vi "ScalarVariantToData.vi"(8 "error in (no error)":errorcluster, 10 "type":T1, 11 "Variant":variant) -> (0 "error out":errorcluster, 2 "Type":string, 3 "Value":string)   [LabVIEW 2019, in "BlueVariantView.lvlib"]
uses:
  BlueVariantView.lvlib
  <vilib>/Utility/Data Type/Type Definitions/Data Type.ctl
  <vilib>/Utility/error.llb/Error Cluster From Error Code.vi
  <vilib>/ErrorRing/Error Ring.xnode
  <vilib>/Utility/Data Type/NI_Data Type.lvlib
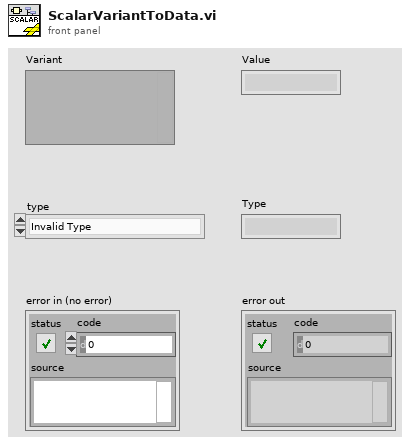
[diagram p1: front panel]
types:
  T1 = typedef "NI_Data Type.lvlib/Data Type.ctl" = enum8{"Invalid Type", "Void", "I8", "I16", "I32", "I64", "U8", "U16", "U32", "U64", "Single Float", "Double Float", "Extended Float", "Single Complex", "Double Complex", "Extended Complex", "Enum U8", "Enum U16", "Enum U32", "Enum U64", "Single Float With Unit", "Double Float With Unit", "Extended Float With Unit", "Single Complex with Unit", "Double Complex with Unit", "Extended Complex with Unit", "Boolean", "String", "Path", "Picture", "Tag", "Array", "Cluster", "Variant", "LV Variant", "Waveform", "Timestamp", "Digital Waveform", "Digital Data", "ExpressData", "Refnum", "External Data", "VI", "Poly VI", "LabVIEW Class Instance", "Fixed Point", "Set Collection", "Map Collection"}
  T2 = typedef "Physical Units__ogtk.ctl" = cluster{"Base Units":enum16{"radian", "steradian", "second", "meter", "kilogram", "ampere", "kelvin", "mole", "candela"}, "Exponent":i16}
  T3 = enum16{"radian", "steradian", "second", "meter", "kilogram", "ampere", "kelvin", "mole", "candela"}
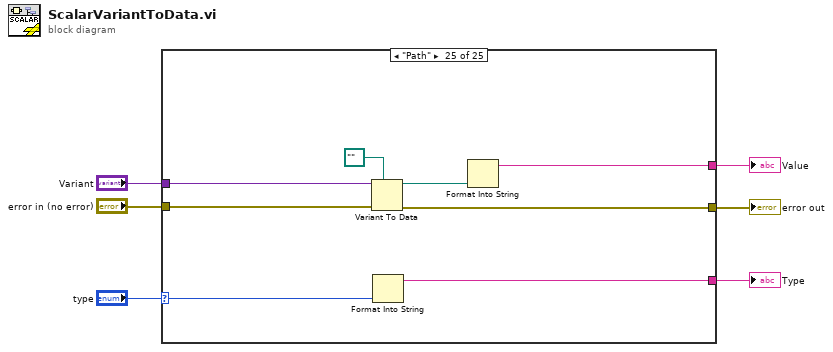
[diagram p0: block diagram]
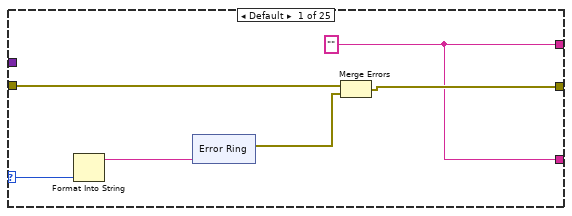
[diagram p2: hidden frame]
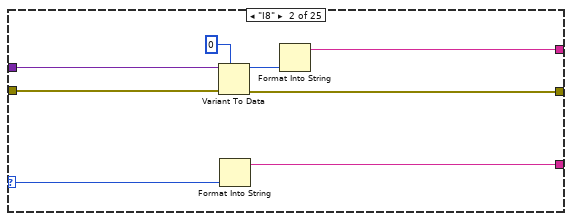
[diagram p3: hidden frame]
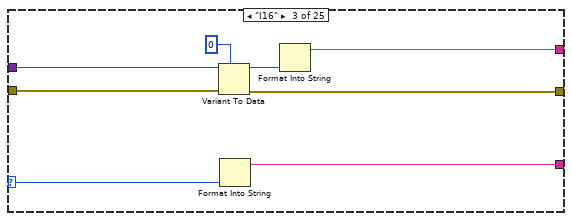
[diagram p4: hidden frame]
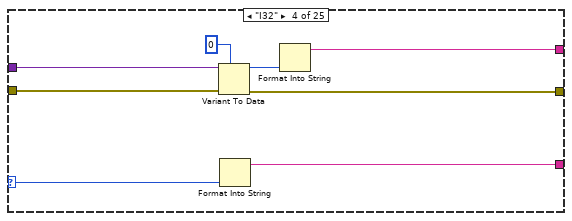
[diagram p5: hidden frame]
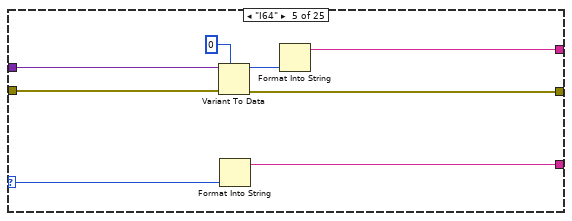
[diagram p6: hidden frame]
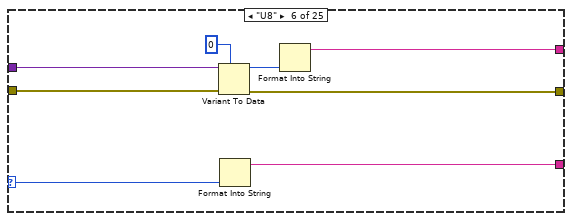
[diagram p7: hidden frame]
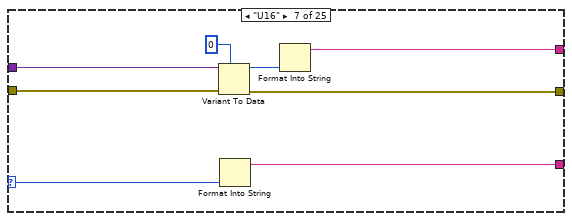
[diagram p8: hidden frame]
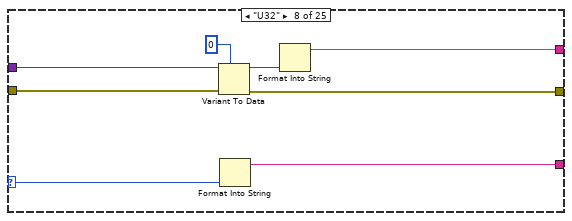
[diagram p9: hidden frame]
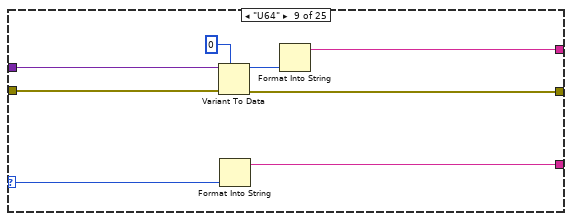
[diagram p10: hidden frame]
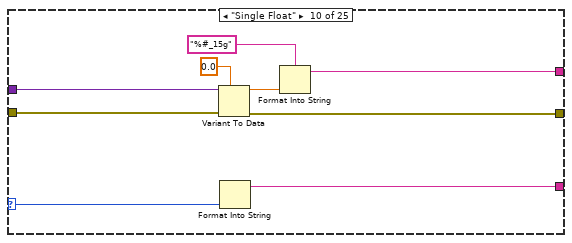
[diagram p11: hidden frame]
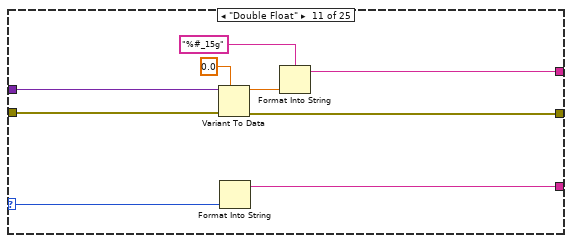
[diagram p12: hidden frame]
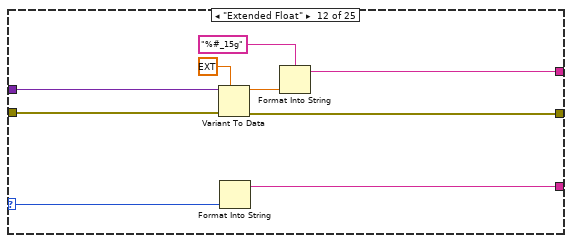
[diagram p13: hidden frame]
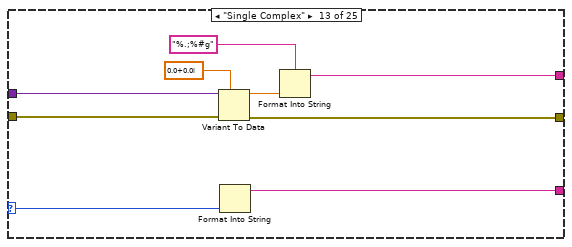
[diagram p14: hidden frame]
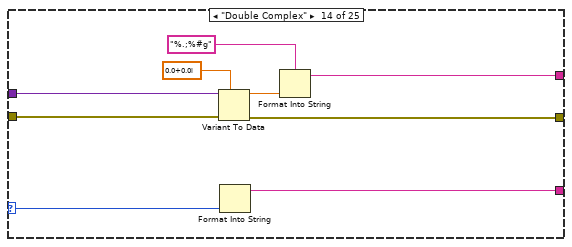
[diagram p15: hidden frame]
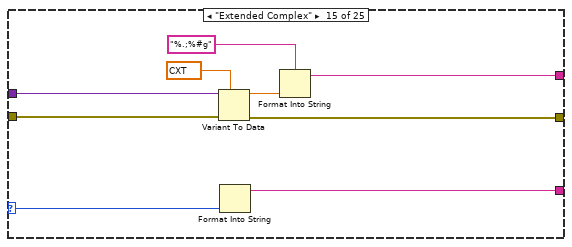
[diagram p16: hidden frame]
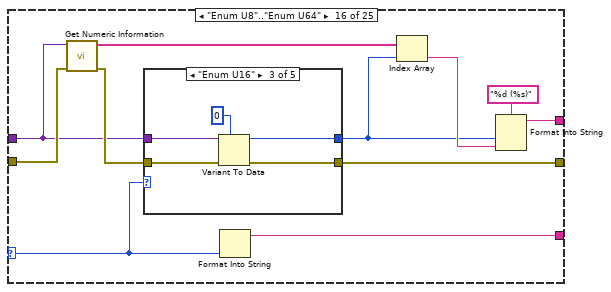
[diagram p17: hidden frame]
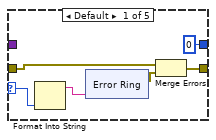
[diagram p18: hidden frame]
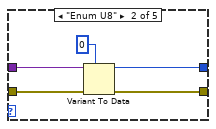
[diagram p19: hidden frame]
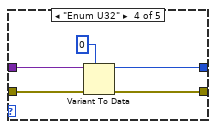
[diagram p20: hidden frame]
diagram:
  n1 = case shown="\"Path\"" "type" {
    selector: "type" -> [w12 w23 w31 w39 w47 w55 w63 w71 w79 w88 w97 w106 w115 w124 w133 w142 w192 w205 w218 w231 w244 w257 w264 w271 w279]
    tunnel: "Variant" -> [_ w27 w35 w43 w51 w59 w67 w75 w83 w92 w101 w110 w119 w128 w137 w143 w185 w198 w211 w224 w237 w250 w267 w274 w282]
    tunnel: "error in (no error)" -> [w10 w26 w34 w42 w50 w58 w66 w74 w82 w91 w100 w109 w118 w127 w136 w145 w187 w200 w213 w226 w239 w252 w266 w273 w281]
    tunnel: [w8 w24 w32 w40 w48 w56 w64 w72 w80 w89 w98 w107 w116 w125 w134 w148 w193 w206 w219 w232 w245 w258 w265 w272 w280] -> w4
    tunnel: [w7 w22 w30 w38 w46 w54 w62 w70 w78 w87 w96 w105 w114 w123 w132 w147 w191 w204 w217 w230 w243 w256 w263 w270 w278] -> w2
    tunnel: [w7 w20 w28 w36 w44 w52 w60 w68 w76 w85 w94 w103 w112 w121 w130 w146 w189 w202 w215 w228 w241 w254 w261 w268 w275] -> w1
    frame Default {
      w7 = ""
      n2 = Format Into String(w12) -> (resulting string=w11:string)  [unwired: 3 in, 1 out]
      n3 = xnode "Error Ring"("parameter 0"=w11) -> ("error out"=w9:errorcluster)
      n4 = Merge Errors(w10, w9) -> (w8:errorcluster)
    }
    frame "I8" {
      n5 = Variant To Data(error in=w26, type=i8 0, Variant=w27) -> (data=w21:i8, error out=w24:errorcluster)
      n6 = Format Into String(w23) -> (resulting string=w22:string)  [unwired: 3 in, 1 out]
      n7 = Format Into String(w21) -> (resulting string=w20:string)  [unwired: 3 in, 1 out]
    }
    frame "I16" {
      n8 = Variant To Data(error in=w34, type=i16 0, Variant=w35) -> (data=w29:i16, error out=w32:errorcluster)
      n9 = Format Into String(w31) -> (resulting string=w30:string)  [unwired: 3 in, 1 out]
      n10 = Format Into String(w29) -> (resulting string=w28:string)  [unwired: 3 in, 1 out]
    }
    frame "I32" {
      n11 = Variant To Data(error in=w42, type=0, Variant=w43) -> (data=w37:i32, error out=w40:errorcluster)
      n12 = Format Into String(w39) -> (resulting string=w38:string)  [unwired: 3 in, 1 out]
      n13 = Format Into String(w37) -> (resulting string=w36:string)  [unwired: 3 in, 1 out]
    }
    frame "I64" {
      n14 = Variant To Data(error in=w50, type=i64 0, Variant=w51) -> (data=w45:i64, error out=w48:errorcluster)
      n15 = Format Into String(w47) -> (resulting string=w46:string)  [unwired: 3 in, 1 out]
      n16 = Format Into String(w45) -> (resulting string=w44:string)  [unwired: 3 in, 1 out]
    }
    frame "U8" {
      n17 = Variant To Data(error in=w58, type=u8 0, Variant=w59) -> (data=w53:u8, error out=w56:errorcluster)
      n18 = Format Into String(w55) -> (resulting string=w54:string)  [unwired: 3 in, 1 out]
      n19 = Format Into String(w53) -> (resulting string=w52:string)  [unwired: 3 in, 1 out]
    }
    frame "U16" {
      n20 = Variant To Data(error in=w66, type=u16 0, Variant=w67) -> (data=w61:u16, error out=w64:errorcluster)
      n21 = Format Into String(w63) -> (resulting string=w62:string)  [unwired: 3 in, 1 out]
      n22 = Format Into String(w61) -> (resulting string=w60:string)  [unwired: 3 in, 1 out]
    }
    frame "U32" {
      n23 = Variant To Data(error in=w74, type=u32 0, Variant=w75) -> (data=w69:u32, error out=w72:errorcluster)
      n24 = Format Into String(w71) -> (resulting string=w70:string)  [unwired: 3 in, 1 out]
      n25 = Format Into String(w69) -> (resulting string=w68:string)  [unwired: 3 in, 1 out]
    }
    frame "U64" {
      n26 = Variant To Data(error in=w82, type=u64 0, Variant=w83) -> (data=w77:u64, error out=w80:errorcluster)
      n27 = Format Into String(w79) -> (resulting string=w78:string)  [unwired: 3 in, 1 out]
      n28 = Format Into String(w77) -> (resulting string=w76:string)  [unwired: 3 in, 1 out]
    }
    frame "Single Float" {
      n29 = Variant To Data(error in=w91, type=sgl 0.0, Variant=w92) -> (data=w86:sgl, error out=w89:errorcluster)
      n30 = Format Into String(w88) -> (resulting string=w87:string)  [unwired: 3 in, 1 out]
      n31 = Format Into String(format string="%#_15g", w86) -> (resulting string=w85:string)  [unwired: 2 in, 1 out]
    }
    frame "Double Float" {
      n32 = Variant To Data(error in=w100, type=0.0, Variant=w101) -> (data=w95:dbl, error out=w98:errorcluster)
      n33 = Format Into String(w97) -> (resulting string=w96:string)  [unwired: 3 in, 1 out]
      n34 = Format Into String(format string="%#_15g", w95) -> (resulting string=w94:string)  [unwired: 2 in, 1 out]
    }
    frame "Extended Float" {
      n35 = Variant To Data(error in=w109, type=ext 0.0, Variant=w110) -> (data=w104:ext, error out=w107:errorcluster)
      n36 = Format Into String(w106) -> (resulting string=w105:string)  [unwired: 3 in, 1 out]
      n37 = Format Into String(format string="%#_15g", w104) -> (resulting string=w103:string)  [unwired: 2 in, 1 out]
    }
    frame "Single Complex" {
      n38 = Variant To Data(error in=w118, type=csg 0.0+0.0i, Variant=w119) -> (data=w113:csg, error out=w116:errorcluster)
      n39 = Format Into String(w115) -> (resulting string=w114:string)  [unwired: 3 in, 1 out]
      n40 = Format Into String(format string="%.;%#g", w113) -> (resulting string=w112:string)  [unwired: 2 in, 1 out]
    }
    frame "Double Complex" {
      n41 = Variant To Data(error in=w127, type=cdb 0.0+0.0i, Variant=w128) -> (data=w122:cdb, error out=w125:errorcluster)
      n42 = Format Into String(w124) -> (resulting string=w123:string)  [unwired: 3 in, 1 out]
      n43 = Format Into String(format string="%.;%#g", w122) -> (resulting string=w121:string)  [unwired: 2 in, 1 out]
    }
    frame "Extended Complex" {
      n44 = Variant To Data(error in=w136, type=cxt 0.0+0.0i, Variant=w137) -> (data=w131:cxt, error out=w134:errorcluster)
      n45 = Format Into String(w133) -> (resulting string=w132:string)  [unwired: 3 in, 1 out]
      n46 = Format Into String(format string="%.;%#g", w131) -> (resulting string=w130:string)  [unwired: 2 in, 1 out]
    }
    frame "Enum U8".."Enum U64" {
      n47 = call <vilib>:"Get Numeric Information.vi"("error in (no error)"=w145, "variant"=w143) -> ("error out"=w144:errorcluster, "enum names"=w141:string[])  [unwired: 6 in, 2 out]
      n48 = case shown="\"Enum U16\"" w142 {
        selector: w142 -> [w153 _ _ _ _]
        tunnel: [w150 w165 w170 w175 w180] -> w148
        tunnel: [u64 0 w164 w169 w174 w179] -> w138
        tunnel: w144 -> [w151 w163 w168 w173 w178]
        tunnel: w143 -> [_ w162 w167 w172 w177]
        frame Default {
          n49 = Format Into String(w153) -> (resulting string=w152:string)  [unwired: 3 in, 1 out]
          n50 = xnode "Error Ring"("parameter 0"=w152) -> ("error out"=w149:errorcluster)
          n51 = Merge Errors(w151, w149) -> (w150:errorcluster)
        }
        frame "Enum U8" {
          n52 = Variant To Data(error in=w163, type=u8 0, Variant=w162) -> (data=w164:u8, error out=w165:errorcluster)
        }
        frame "Enum U16" {
          n53 = Variant To Data(error in=w168, type=u16 0, Variant=w167) -> (data=w169:u16, error out=w170:errorcluster)
        }
        frame "Enum U32" {
          n54 = Variant To Data(error in=w173, type=u32 0, Variant=w172) -> (data=w174:u32, error out=w175:errorcluster)
        }
        frame "Enum U64" {
          n55 = Variant To Data(error in=w178, type=u64 0, Variant=w177) -> (data=w179:u64, error out=w180:errorcluster)
        }
      }
      n56 = Format Into String(w142) -> (resulting string=w147:string)  [unwired: 3 in, 1 out]
      n57 = Index Array(array=w141, index=w138) -> (element=w139:string)
      n58 = Format Into String(format string="%d (%s)", w138, w139) -> (resulting string=w146:string)  [unwired: 2 in, 1 out]
    }
    frame "Single Float With Unit" {
      n59 = call <userlib>:"Get Physical Units__ogtk.vi"("error in (no error)"=w187, "Float or Array of Floats"=w185) -> ("error out"=w186:errorcluster, "Physical Units"=w184:T2[])  [unwired: 8 in]
      n60 = Index Array(array=w184) -> (element=w183:T2)  [unwired: 1 in]
      n61 = Variant To Data(error in=w186, type=sgl 0.0, Variant=w185) -> (data=w190:sgl, error out=w193:errorcluster)
      n62 = Format Into String(w192) -> (resulting string=w191:string)  [unwired: 3 in, 1 out]
      n63 = Unbundle By Name(w183) -> ("Base Units"=w182:T3)
      n64 = Format Into String(format string="%#_15g (%s)", w190, w182) -> (resulting string=w189:string)  [unwired: 2 in, 1 out]
    }
    frame "Double Float With Unit" {
      n65 = call <userlib>:"Get Physical Units__ogtk.vi"("error in (no error)"=w200, "Float or Array of Floats"=w198) -> ("error out"=w199:errorcluster, "Physical Units"=w197:T2[])  [unwired: 8 in]
      n66 = Index Array(array=w197) -> (element=w196:T2)  [unwired: 1 in]
      n67 = Variant To Data(error in=w199, type=0.0, Variant=w198) -> (data=w203:dbl, error out=w206:errorcluster)
      n68 = Format Into String(w205) -> (resulting string=w204:string)  [unwired: 3 in, 1 out]
      n69 = Unbundle By Name(w196) -> ("Base Units"=w195:T3)
      n70 = Format Into String(format string="%#_15g (%s)", w203, w195) -> (resulting string=w202:string)  [unwired: 2 in, 1 out]
    }
    frame "Extended Float With Unit" {
      n71 = call <userlib>:"Get Physical Units__ogtk.vi"("error in (no error)"=w213, "Float or Array of Floats"=w211) -> ("error out"=w212:errorcluster, "Physical Units"=w210:T2[])  [unwired: 8 in]
      n72 = Index Array(array=w210) -> (element=w209:T2)  [unwired: 1 in]
      n73 = Variant To Data(error in=w212, type=ext 0.0, Variant=w211) -> (data=w216:ext, error out=w219:errorcluster)
      n74 = Format Into String(w218) -> (resulting string=w217:string)  [unwired: 3 in, 1 out]
      n75 = Unbundle By Name(w209) -> ("Base Units"=w208:T3)
      n76 = Format Into String(format string="%#_15g (%s)", w216, w208) -> (resulting string=w215:string)  [unwired: 2 in, 1 out]
    }
    frame "Single Complex with Unit" {
      n77 = call <userlib>:"Get Physical Units__ogtk.vi"("error in (no error)"=w226, "Float or Array of Floats"=w224) -> ("error out"=w225:errorcluster, "Physical Units"=w223:T2[])  [unwired: 8 in]
      n78 = Index Array(array=w223) -> (element=w222:T2)  [unwired: 1 in]
      n79 = Variant To Data(error in=w225, type=csg 0.0+0.0i, Variant=w224) -> (data=w229:csg, error out=w232:errorcluster)
      n80 = Format Into String(w231) -> (resulting string=w230:string)  [unwired: 3 in, 1 out]
      n81 = Unbundle By Name(w222) -> ("Base Units"=w221:T3)
      n82 = Format Into String(format string="%.;%#g (%s)", w229, w221) -> (resulting string=w228:string)  [unwired: 2 in, 1 out]
    }
    frame "Double Complex with Unit" {
      n83 = call <userlib>:"Get Physical Units__ogtk.vi"("error in (no error)"=w239, "Float or Array of Floats"=w237) -> ("error out"=w238:errorcluster, "Physical Units"=w236:T2[])  [unwired: 8 in]
      n84 = Index Array(array=w236) -> (element=w235:T2)  [unwired: 1 in]
      n85 = Variant To Data(error in=w238, type=cdb 0.0+0.0i, Variant=w237) -> (data=w242:cdb, error out=w245:errorcluster)
      n86 = Format Into String(w244) -> (resulting string=w243:string)  [unwired: 3 in, 1 out]
      n87 = Unbundle By Name(w235) -> ("Base Units"=w234:T3)
      n88 = Format Into String(format string="%.;%#g (%s)", w242, w234) -> (resulting string=w241:string)  [unwired: 2 in, 1 out]
    }
    frame "Extended Complex with Unit" {
      n89 = call <userlib>:"Get Physical Units__ogtk.vi"("error in (no error)"=w252, "Float or Array of Floats"=w250) -> ("error out"=w251:errorcluster, "Physical Units"=w249:T2[])  [unwired: 8 in]
      n90 = Index Array(array=w249) -> (element=w248:T2)  [unwired: 1 in]
      n91 = Variant To Data(error in=w251, type=cxt 0.0+0.0i, Variant=w250) -> (data=w255:cxt, error out=w258:errorcluster)
      n92 = Format Into String(w257) -> (resulting string=w256:string)  [unwired: 3 in, 1 out]
      n93 = Unbundle By Name(w248) -> ("Base Units"=w247:T3)
      n94 = Format Into String(format string="%.;%#g (%s)", w255, w247) -> (resulting string=w254:string)  [unwired: 2 in, 1 out]
    }
    frame "Boolean" {
      n95 = Variant To Data(error in=w266, type=FALSE, Variant=w267) -> (data=w262:bool, error out=w265:errorcluster)
      n96 = Format Into String(w264) -> (resulting string=w263:string)  [unwired: 3 in, 1 out]
      n97 = Format Into String(w262) -> (resulting string=w261:string)  [unwired: 3 in, 1 out]
    }
    frame "String" {
      n98 = Variant To Data(error in=w273, type="", Variant=w274) -> (data=w268:string, error out=w272:errorcluster)
      n99 = Format Into String(w271) -> (resulting string=w270:string)  [unwired: 3 in, 1 out]
    }
    frame "Path" {
      n100 = Variant To Data(error in=w281, type=path "", Variant=w282) -> (data=w276:path, error out=w280:errorcluster)
      n101 = Format Into String(w279) -> (resulting string=w278:string)  [unwired: 3 in, 1 out]
      n102 = Format Into String(w276) -> (resulting string=w275:string)  [unwired: 3 in, 1 out]
    }
  }
  "error out" <- w4
  "Value" <- w1
  "Type" <- w2
